vi "Index the Displayed Data_Ctrls-某型振动实验台测试系统.vi"(6 "Results":T1, 10 "Channel Info":T2=[{"Color"=0, "channel"=0}, {"Color"=0, "channel"=0}, {"Color"=0, "channel"=0}, {"Color"=0, "channel"=0}, {"Color"=0, "channel"=0}], 11 "DataIn":waveform(dbl)[](array[waveform])) -> (2 "IndexData":waveform(dbl)[](array[waveform])=[{"t0"=timestamp(0 s since 1904-01-01), "dt"=1.0, "Y"=[]}, {"t0"=timestamp(0 s since 1904-01-01), "dt"=1.0, "Y"=[]}, {"t0"=timestamp(0 s since 1904-01-01), "dt"=1.0, "Y"=[]}], 3 "Dis Result":T1, 4 "Color Array":u32[](array[numeric]))   [LabVIEW 2011]
doc: "索引出需要显示在前面板上的波形数据、分析结果数组以及各波形的颜色数组。"
panel:
  in  "Data Initialize":waveform(dbl)[](array[waveform])
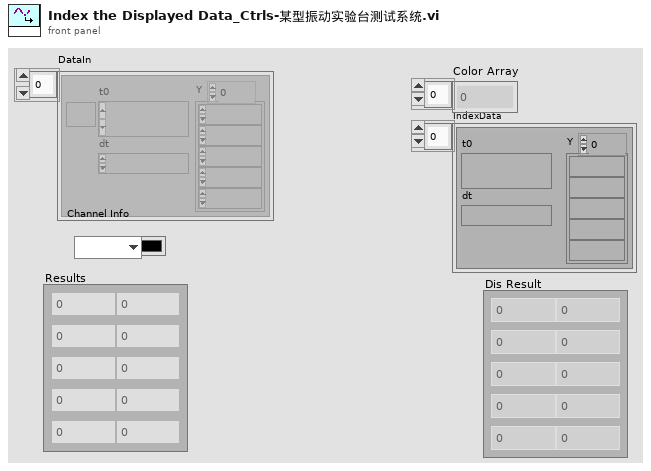
[diagram p1: front panel]
types:
  T1 = typedef "Display Information_Ctrls-某型振动实验台测试系统.ctl" = cluster{"Frequency":dbl, "RMS":dbl}[]
  T2 = typedef "Channel Selection_Ctrls-某型振动实验台测试系统.ctl" = cluster{"Color":u32, "channel":u16}[]
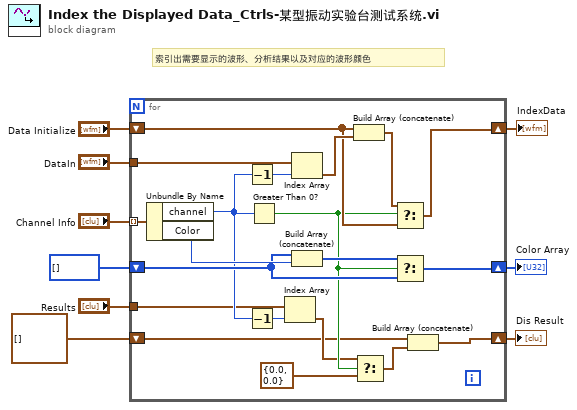
[diagram p0: block diagram]
diagram:
  # "索引出需要显示的波形、分析结果以及对应的波形颜色"
  n1 = for {
    tunnel: "Channel Info" -> [w29] mode=indexing
    shift-right: [w24] -> w9
    shift-left: "Data Initialize" -> [w25]
    tunnel: "DataIn" -> [w28]
    shift-right: [w20] -> w2
    shift-left: u32[] [] -> [w21]
    tunnel: "Results" -> [w16]
    shift-right: [w10] -> w1
    shift-left: T1 [] ("Display Info") -> [w11]
    n2 = Unbundle By Name(w29) -> ("channel"=w17:u16, "Color"=w23:u32)
    n3 = Decrement(x=w17) -> (x-1=w19:u16)
    n4 = Decrement(x=w17) -> (x-1=w15:u16)
    n5 = Greater Than 0?(x=w17) -> (x > 0?=w18:bool)
    n6 = Index Array(array=w16, index=w15) -> (element=w14:cluster{"Frequency":dbl, "RMS":dbl})
    n7 = Index Array(array=w28, index=w19) -> (element=w27:waveform(dbl))
    n8 = Build Array (concatenate)(w21, w23) -> (w22:u32[])
    n9 = Build Array (concatenate)(w25, w27) -> (w26:waveform(dbl)[])
    n10 = Select(t=w14, s=w18, f=cluster{"Frequency":dbl, "RMS":dbl} {"Frequency"=0.0, "RMS"=0.0}) -> (s? t:f=w12:cluster{"Frequency":dbl, "RMS":dbl})
    n11 = Select(t=w26, s=w18, f=w25) -> (s? t:f=w24:waveform(dbl)[])
    n12 = Select(t=w22, s=w18, f=w21) -> (s? t:f=w20:u32[])
    n13 = Build Array (concatenate)(w11, w12) -> (w10:T1)
  }
  "IndexData" <- w9
  "Color Array" <- w2
  "Dis Result" <- w1
